vi "Close Client Context.vi"(8 "error in (no error)":errorcluster, 11 "ContextID":T1) -> (0 "error out":errorcluster)   [LabVIEW 2019, in "grpc-lvsupport.lvlib"]
uses:
  grpc-lvsupport.lvlib
  Shared/grpcId.ctl
  <vilib>/Utility/error.llb/Error Cluster From Error Code.vi
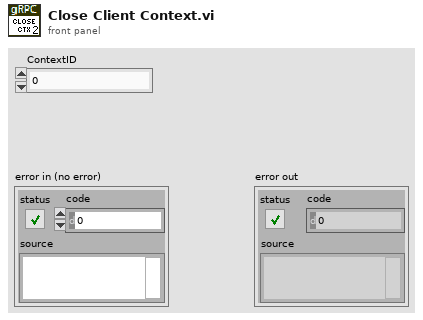
[diagram p1: front panel]
types:
  T1 = typedef "grpc-lvsupport.lvlib/grpcId.ctl" = u64
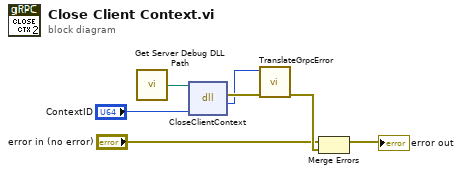
[diagram p0: block diagram]
diagram:
  n1 = call "Get Server Debug DLL Path.vi"() -> ("Server Debug DLL Path"=w6:path)
  n2 = dll-call lib="?" fn="CloseClientContext"(path in=w6, "contextId"="ContextID") -> (error out=w7:errorcluster, "return type"=w5:i32)  [unwired: 3 in, 1 out]
  n3 = call "TranslateGrpcError.vi"("error in"=w7, "Error Code"=w5) -> ("error out"=w4:errorcluster)  [unwired: 9 in]
  n4 = Merge Errors("error in (no error)", w4) -> (→"error out":errorcluster)
